vi "4.7.vi"() -> ()   [LabVIEW 2017]
panel:
  out "猜测次数":i32
  out "随机数":i32
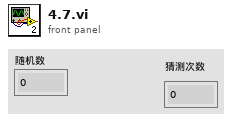
[diagram p1: front panel]
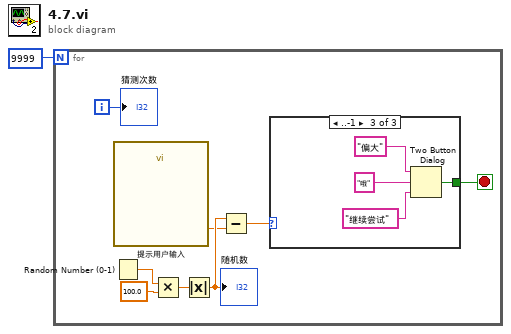
[diagram p0: block diagram]
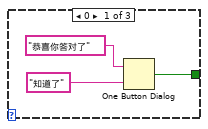
[diagram p2: hidden frame]
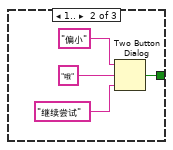
[diagram p3: hidden frame]
diagram:
  n1 = for {
    N: 9999 -> [_]
    i -> [w4]
    stop <- w3 stop-if-true
    n2 = Random Number (0-1)() -> (number: 0 to 1=w9:dbl)
    n3 = call "提示用户输入"() -> ("请在1-1000猜"=w2:dbl)  [unwired: 17 in, 2 out]
    n4 = Multiply(x=w9, y=100.0) -> (x*y=w7:dbl)
    n5 = Absolute Value(x=w7) -> (abs(x)=w6:dbl)
    "随机数" <- w6
    n6 = Subtract(x=w6, y=w2) -> (x-y=w5:dbl)
    n7 = case shown="..-1" w5 {
      tunnel: [w12 w13 w17] -> w3
      frame 0 {
        n8 = One Button Dialog(message="恭喜你答对了", button name ("OK")="知道了") -> (true=w12:bool)
      }
      frame 1.. {
        n9 = Two Button Dialog(message="偏小", 1:"继续尝试", 2:"哦") -> (T button?=w13:bool)
      }
      frame ..-1 {
        n10 = Two Button Dialog(message="偏大", 1:"继续尝试", 2:"哦") -> (T button?=w17:bool)
      }
    }
    "猜测次数" <- w4
  }
